vi "MessageCommands.vi"(11 "Robot":T1={"id"=0, "function"=enum."Attacker", "x"=0.0, "y"=0.0, "orientation"=0.0, "v_tangent"=0.0, "v_normal"=0.0, "v_ang"=0.0, "kick_x"=0.0, "kick_z"=0.0, "dribble"=FALSE, "Timestamp"=timestamp(0 s since 1904-01-01), "estimatives"={"est_v_tangent"=0.0, "est_v_normal"=0.0, "est_vx"=0.0, "est_vy"=0.0, "Pos Robot Est"=[]}, "dest_x_kick"=0.0, "dest_y_kick"=0.0, "Gap Coord"=[], "States"=enum."GoToTangent", "Path "=[], "Path  Smooth"=[], "Dest"=[], "vx_desired"=0.0, "vy_desired"=0.0, "slowBehavior"=FALSE, "VSSStates"=enum."Pass"}) -> (1 "Array":u8[](array[numeric]))   [LabVIEW 2023]
uses:
  Vision_class/Old vision/Controls/AI Robot.ctl
  Vision_class/Old vision/Controls/Functions Enum.ctl
  Vision_class/Old vision/Controls/AttackerStates.ctl
  Vision_class/Old vision/Controls/PathDests.ctl
  Vision_class/Old vision/Controls/PathDest.ctl
  Game_class/Navigation/VSSNavigation/VSSAttackerStates.ctl
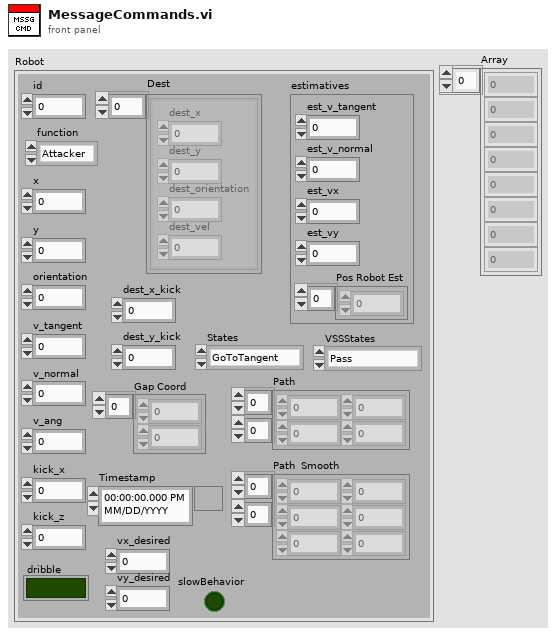
[diagram p1: front panel]
types:
  T1 = typedef "AI Robot.ctl" = cluster{"id":u32, "function":T2, "x":dbl, "y":dbl, "orientation":dbl, "v_tangent":dbl, "v_normal":dbl, "v_ang":dbl, "kick_x":dbl, "kick_z":dbl, "dribble":bool, "Timestamp":timestamp, "estimatives":cluster{"est_v_tangent":dbl, "est_v_normal":dbl, "est_vx":dbl, "est_vy":dbl, "Pos Robot Est":dbl[]}, "dest_x_kick":dbl, "dest_y_kick":dbl, "Gap Coord":dbl[], "States":T3, "Path ":dbl[][], "Path  Smooth":dbl[][], "Dest":T4, "vx_desired":dbl, "vy_desired":dbl, "slowBehavior":bool, "VSSStates":T6}
  T2 = typedef "Functions Enum.ctl" = enum16{"2nd Striker", "Attacker", "Goalie", "Defender", "Striker", "Goto 0", "Dummy", "Kicker", "ZigZag 0", "ZigZag 1", "ZigZag 2", "ZigZag 3", "ZigZag 4", "ZigZag 5", "ZigZag 6", "ZigZag 7", "ZigZag 8", ""}
  T3 = typedef "AttackerStates.ctl" = enum16{"Pass", "GoToTangent", "BallGetting", "GoToKick", ""}
  T4 = typedef "PathDests.ctl" = T5[]
  T5 = typedef "PathDest.ctl" = cluster{"dest_x":dbl, "dest_y":dbl, "dest_orientation":dbl, "dest_vel":dbl}
  T6 = typedef "VSSAttackerStates.ctl" = enum16{"Pass", "GoToTangent", "BallGetting", "GoToKick", "Rotate anti-clockwise", "Rotate Clockwise", ""}
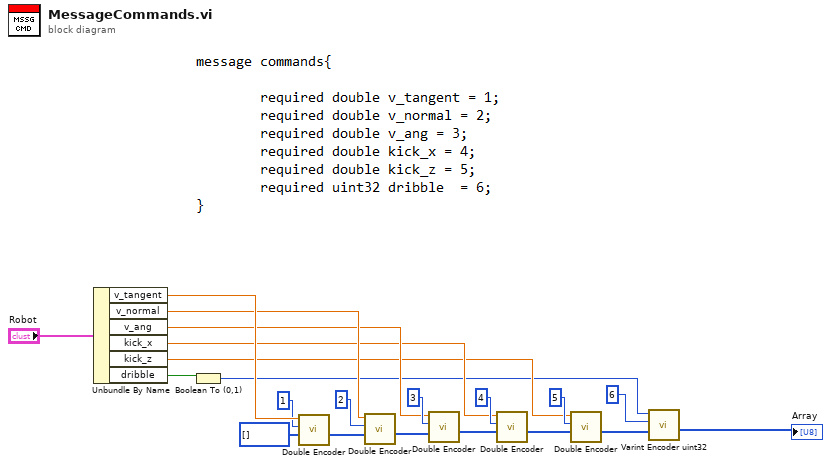
[diagram p0: block diagram]
diagram:
  n1 = Unbundle By Name("Robot") -> ("v_tangent"=w20:dbl, "v_normal"=w10:dbl, "v_ang"=w9:dbl, "kick_x"=w8:dbl, "kick_z"=w7:dbl, "dribble"=w4:bool)
  n2 = Boolean To (0,1)(Boolean=w4) -> (0, 1=w3:i16)
  n3 = call "Double Encoder.vi"("Array In"=u8[] [], "Key"=u32 1, "Value"=w20) -> ("Array"=w17:u8[])  [unwired: 8 in]
  n4 = call "Double Encoder.vi"("Array In"=w17, "Key"=u32 2, "Value"=w10) -> ("Array"=w15:u8[])  [unwired: 8 in]
  n5 = call "Double Encoder.vi"("Array In"=w15, "Key"=u32 3, "Value"=w9) -> ("Array"=w13:u8[])  [unwired: 8 in]
  n6 = call "Double Encoder.vi"("Array In"=w13, "Key"=u32 4, "Value"=w8) -> ("Array"=w11:u8[])  [unwired: 8 in]
  n7 = call "Double Encoder.vi"("Array In"=w11, "Key"=u32 5, "Value"=w7) -> ("Array"=w6:u8[])  [unwired: 8 in]
  n8 = call "Varint Encoder uint32.vi"("Array In"=w6, "Key"=u32 6, "Value"=w3) -> ("Array"=→"Array":u8[])  [unwired: 8 in]
